vi "HanningWindow.vi"(1 "Type":enum16{"Full", "Partial"}(ring), 3 "Array":cdb[](array[numeric]) format="%.2f") -> (0 "output Array":cdb[](array[numeric]) format="%.2f")   [LabVIEW 2012]
uses:
  <vilib>/Analysis/1siggen.llb/Ramp Pattern by Samples.vi
  <vilib>/Analysis/NI_AALBase.lvlib
panel:
  out "Waveform Graph":dbl[](graph)
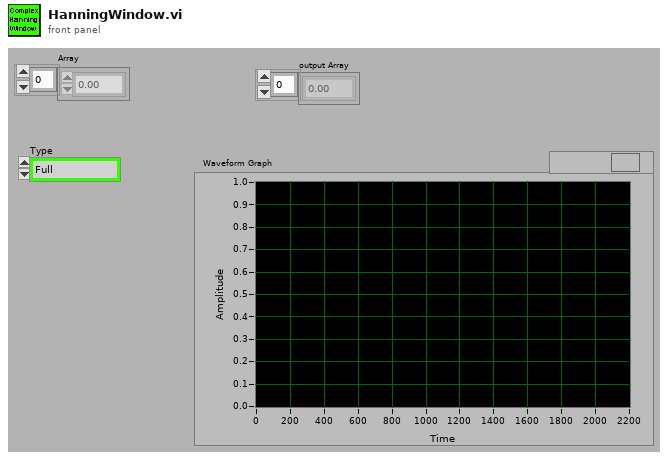
[diagram p1: front panel]
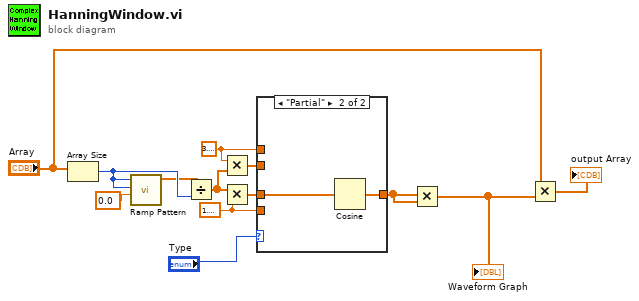
[diagram p0: block diagram]
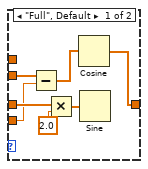
[diagram p2: hidden frame]
diagram:
  w8 = 3.141592653589793
  w6 = 1.5707963267948966
  n1 = Array Size(array="Array") -> (size(s)=w4:i32)
  n2 = call-poly <vilib>:"Ramp Pattern.vi"("start"=0.0, "end"=w4, "samples"=w4) -> ("Ramp Pattern"=w3:dbl[])  [unwired: 7 in, 1 out]
  n3 = Divide(x=w3, y=w4) -> (x/y=w9:dbl[])
  n4 = Multiply(x=w8, y=w9) -> (x*y=w7:dbl[])
  n5 = Multiply(x=w9, y=w6) -> (x*y=w10:dbl[])
  n6 = case shown="\"Partial\"" "Type" {
    tunnel: w10 -> [w19 w21]
    tunnel: [w15 w22] -> w12
    tunnel: w7 -> [w17 _]
    tunnel: w8 -> [_ _]
    tunnel: w6 -> [w14 _]
    frame "Full", Default {
      n7 = Subtract(x=w17, y=w14) -> (x-y=w16:dbl[])
      n8 = Multiply(x=w19, y=2.0) -> (x*y=w20:dbl[])
      n9 = Cosine(x=w16) -> (cos(x)=w15:dbl[])
      n10 = Sine(x=w20) -> ()  [unwired: 1 out]
    }
    frame "Partial" {
      n11 = Cosine(x=w21) -> (cos(x)=w22:dbl[])
    }
  }
  n12 = Multiply(x=w12, y=w12) -> (x*y=w1:dbl[])
  "Waveform Graph" <- w1
  n13 = Multiply(x="Array", y=w1) -> (x*y=→"output Array":cdb[])
